vi "Lockin.Low Pass Filter.vi"(8 "error in (no error)":errorcluster, 11 "Lockin.DAQ":refnum<class "Instrument.DAQ.lvclass">) -> (0 "error out":errorcluster, 3 "Lockin.DAQ":refnum<class "Instrument.DAQ.lvclass">)   [LabVIEW 2019, in "DSP.lvclass"]
uses:
  DSP.lvclass
  Instrument.DAQ/Instrument.DAQ.lvclass
  C:/Program Files (x86)/National Instruments/LabVIEW 2019/vi.lib/JKI/JKI SMO/SMO/SMO.lvclass
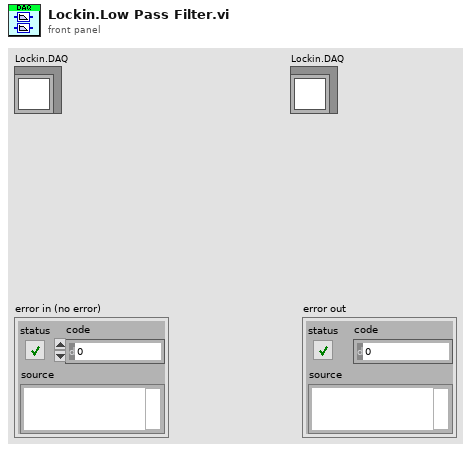
[diagram p1: front panel]
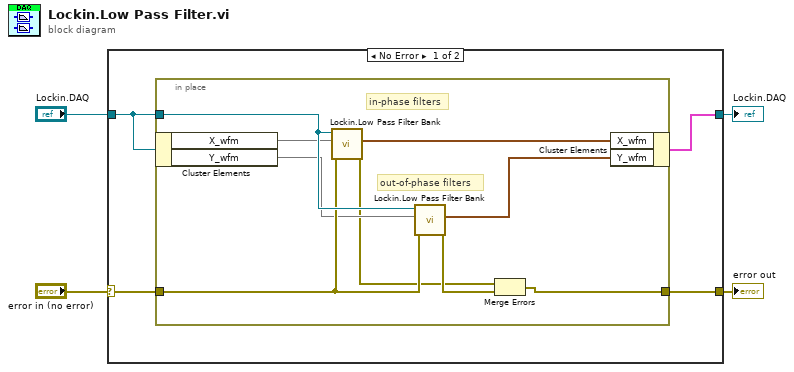
[diagram p0: block diagram]
diagram:
  n1 = case shown="No Error" "error in (no error)" {
    selector: "error in (no error)" -> [w7 w19]
    tunnel: [w8 w19] -> w4
    tunnel: [w5 w18] -> w3
    tunnel: "Lockin.DAQ" -> [w6 w18]
    frame No Error {
      n2 = in-place {
        in-place-border: [w17] -> w8
        in-place-border: w6 -> [w16]
        in-place-border: w7 -> [w15]
        # "out-of-phase filters"
        # "in-phase filters"
        n3 = in-place-cluster #1(w6) -> ("X_wfm"=w14, "Y_wfm"=w13)
        n4 = call "Lockin.Low Pass Filter Bank.vi"("error in (no error)"=w15, "WFms in"=w14, "Instrument.DAQ in"=w16) -> ("error out"=w10:errorcluster, "Wfms out"=w12:waveform(dbl)[])  [unwired: 7 in]
        n5 = call "Lockin.Low Pass Filter Bank.vi"("error in (no error)"=w15, "WFms in"=w13, "Instrument.DAQ in"=w16) -> ("error out"=w11:errorcluster, "Wfms out"=w9:waveform(dbl)[])  [unwired: 7 in]
        n6 = Merge Errors(w10, w11) -> (w17:errorcluster)
        n7 = in-place-cluster #1("X_wfm"=w12, "Y_wfm"=w9) -> (w5:cluster{})
      }
    }
    frame Error {
    }
  }
  "error out" <- w4
  "Lockin.DAQ" <- w3
